vi "ControllerTestBench.vi"() -> ()   [LabVIEW 2016]
uses:
  <vilib>/addons/control/pid/pid.llb/PID (DBL).vi
  <vilib>/addons/Fuzzy Logic/FL Fuzzy Controller (MISO).vi
  <vilib>/addons/control/pid/NI_PID_pid.lvlib
  <vilib>/addons/Fuzzy Logic/NI_Fuzzy_Logic_API.lvlib
  <vilib>/Analysis/NI_AALBase.lvlib
panel:
  out "D":dbl
  out "I":dbl
  out "P":dbl
  out "v":dbl
  in  "RC out":dbl
  out "standard deviation":dbl format="%0.2f"
  out "mean":dbl format="%0.2f"
  out "Array":u32[](array[numeric])
  in  "Controller":enum16{"LQR", "Fuzzy", "P", "PD"}(ring)
  out "Output LQR":dbl
  out "LQR Direction":bool
  out "Fuzzy out":dbl
  in  "K":dbl[](array[numeric]) format="%#_13g"
  in  "Output range  P":cluster{"output high":dbl, "output low":dbl}={"output high"=100.0, "output low"=-100.0} {"output low" format="%.2f"; "output high" format="%.2f"}
  in  "P gains":T1={"Proportional gain (Kc)"=2.0, "Integral time (Ti, min)"=0.0, "Derivative time (Td, min)"=0.0} {"Derivative time (Td, min)" format="%.4f"; "Integral time (Ti, min)" format="%.3f"; "Proportional gain (Kc)" format="%.3f"}
  out "P output":dbl format="%.2f"
  in  "Number of iterations":i32=10000
  in  "Output range  PD":cluster{"output high":dbl, "output low":dbl}={"output high"=100.0, "output low"=-100.0} {"output low" format="%.2f"; "output high" format="%.2f"}
  in  "PD gains":T1={"Proportional gain (Kc)"=2.0, "Integral time (Ti, min)"=0.0, "Derivative time (Td, min)"=0.0} {"Derivative time (Td, min)" format="%.4f"; "Integral time (Ti, min)" format="%.3f"; "Proportional gain (Kc)" format="%.3f"}
  out "PD output":dbl format="%.2f"
  out "Elapsed time(usec)":dbl
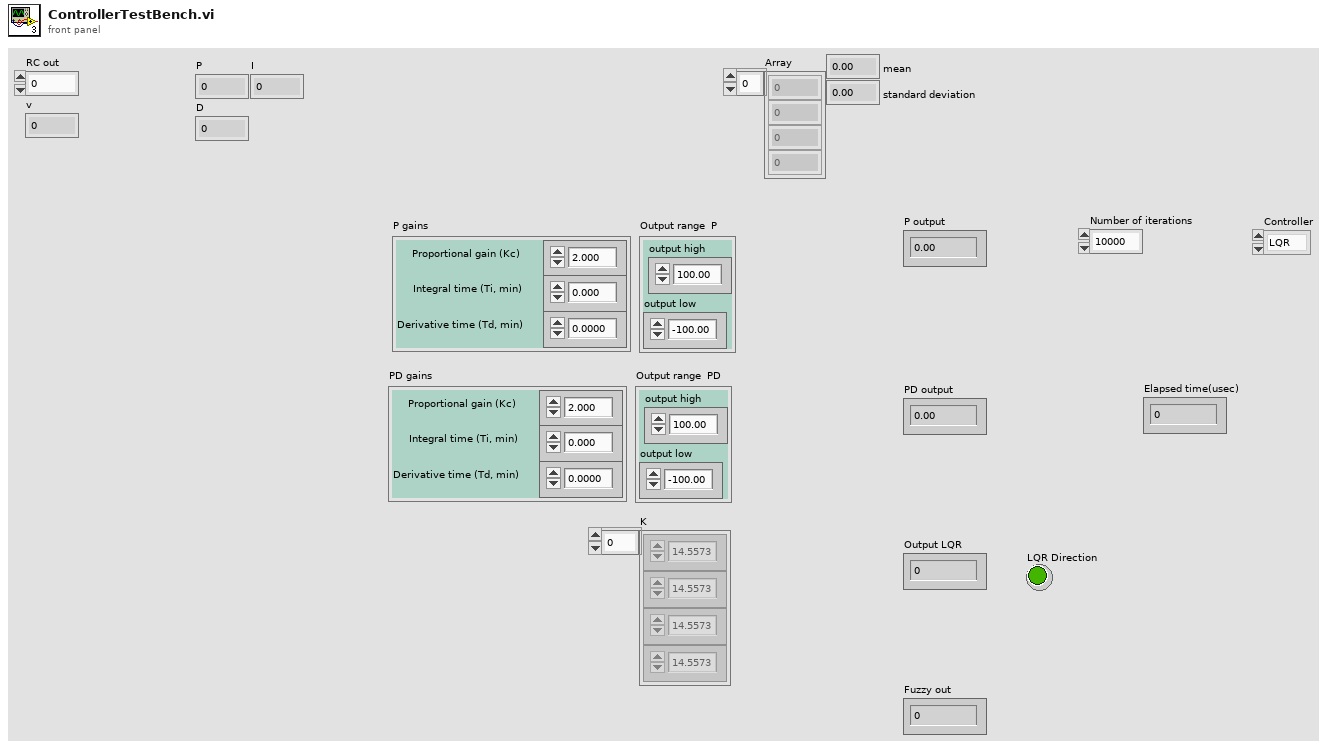
[diagram p1: front panel]
types:
  T1 = cluster{"Proportional gain (Kc)":dbl, "Integral time (Ti, min)":dbl, "Derivative time (Td, min)":dbl}
  T2 = typedef "NI_Fuzzy_Logic_API.lvlib/FL System.ctl" = cluster{"input variables":T3[], "output variables":T3[], "rules":T6[], "defuzzification method":T12, "description":string, "user MF interpolating polynomials":T13[]}
  T3 = typedef "NI_Fuzzy_Logic_API.lvlib/FL Variable.ctl" = cluster{"name":string, "range":dbl[], "MFs":T4[]}
  T4 = typedef "NI_Fuzzy_Logic_API.lvlib/FL Membership Function.ctl" = cluster{"name":string, "shape":T5, "points":dbl[], "color":u32, "user-defined shape index":i32}
  T5 = typedef "NI_Fuzzy_Logic_API.lvlib/FL Membership Function Shape.ctl" = u16
  T6 = typedef "NI_Fuzzy_Logic_API.lvlib/FL Rule.ctl" = cluster{"antecedents":T7[], "antecedent connective":T9, "consequents":T10[], "consequent implication":T11, "degree of support":dbl}
  T7 = typedef "NI_Fuzzy_Logic_API.lvlib/FL Antecedent.ctl" = cluster{"Var Index":i32, "MF Index":i32, "Cond":T8}
  T8 = typedef "NI_Fuzzy_Logic_API.lvlib/FL Modifier.ctl" = u16
  T9 = typedef "NI_Fuzzy_Logic_API.lvlib/FL Antecedent Connective.ctl" = u16
  T10 = typedef "NI_Fuzzy_Logic_API.lvlib/FL Consequent.ctl" = cluster{"Var Index":i32, "MF Index":i32, "Cond":T8}
  T11 = typedef "NI_Fuzzy_Logic_API.lvlib/FL Consequent Implication.ctl" = u16
  T12 = typedef "NI_Fuzzy_Logic_API.lvlib/FL Defuzzification.ctl" = u16
  T13 = typedef "NI_Fuzzy_Logic_API.lvlib/FL Interpolating polynomials.ctl" = cluster{"X":dbl[], "Y":dbl[], "Y(x) coeff":dbl[][], "X(y) coeff":dbl[][], "Area(y) coeff":dbl[][], "coa_x(y) coeff":dbl[][]}
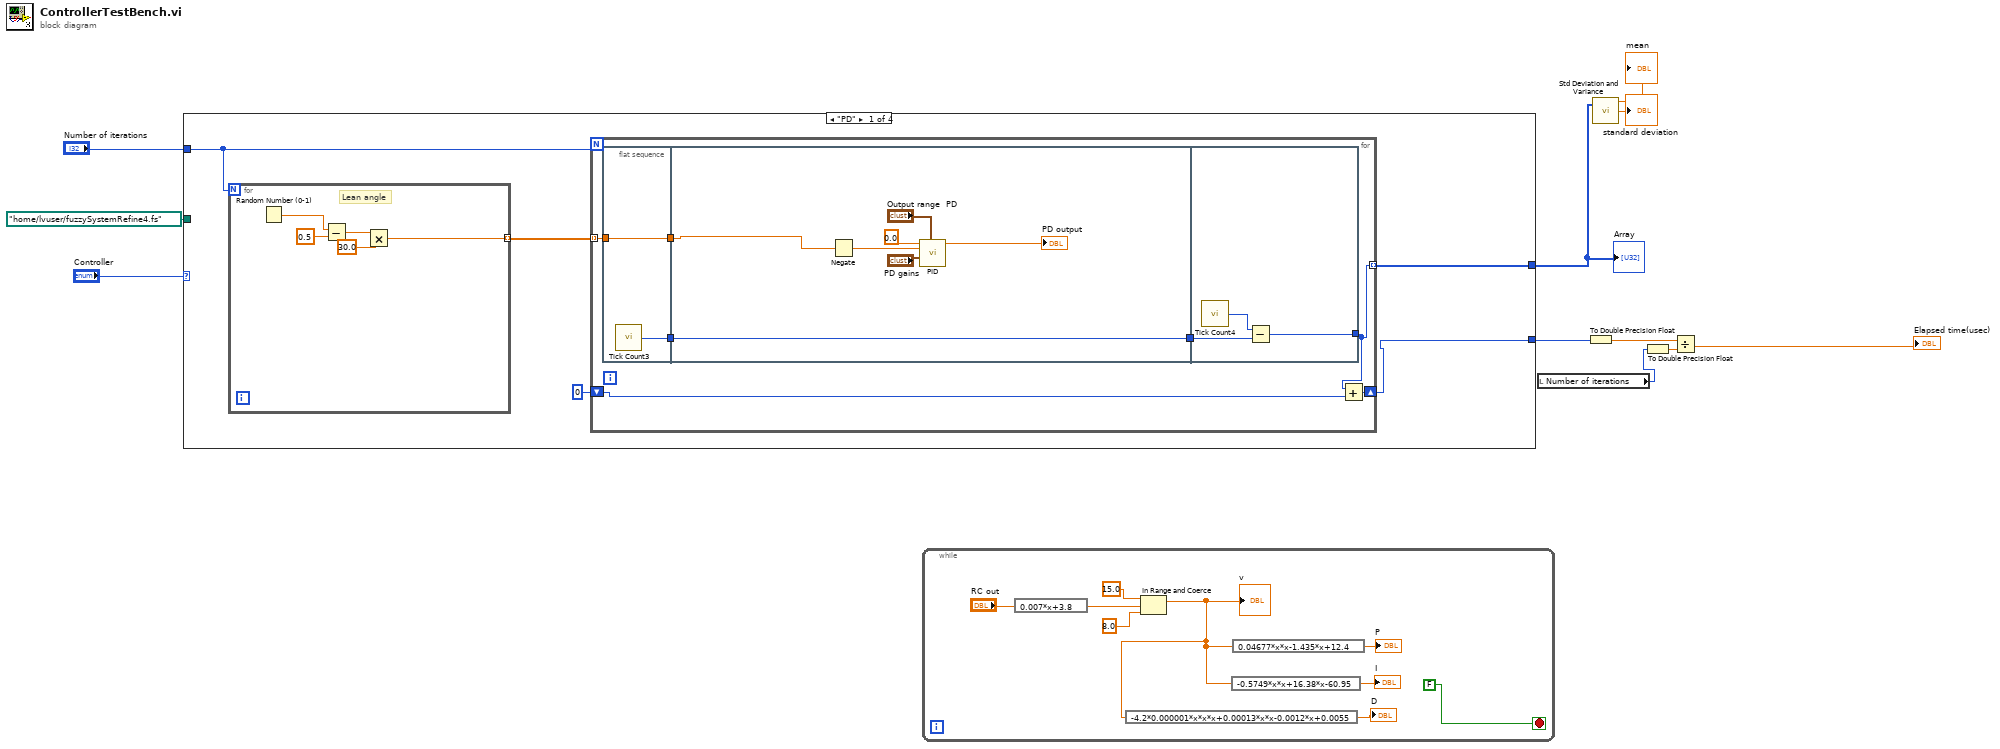
[diagram p0: block diagram]
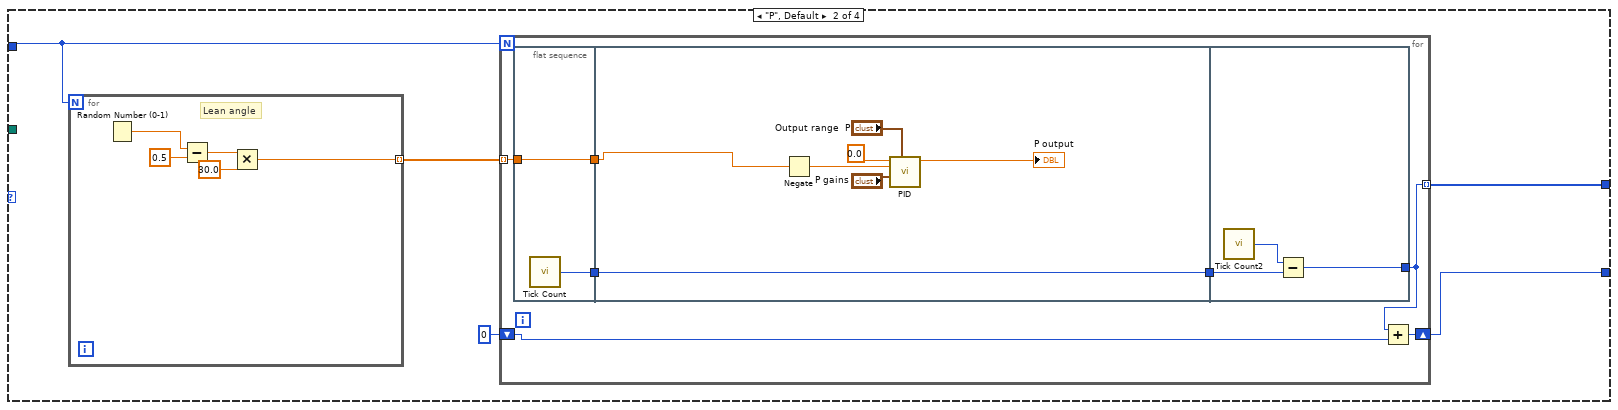
[diagram p2: hidden frame]
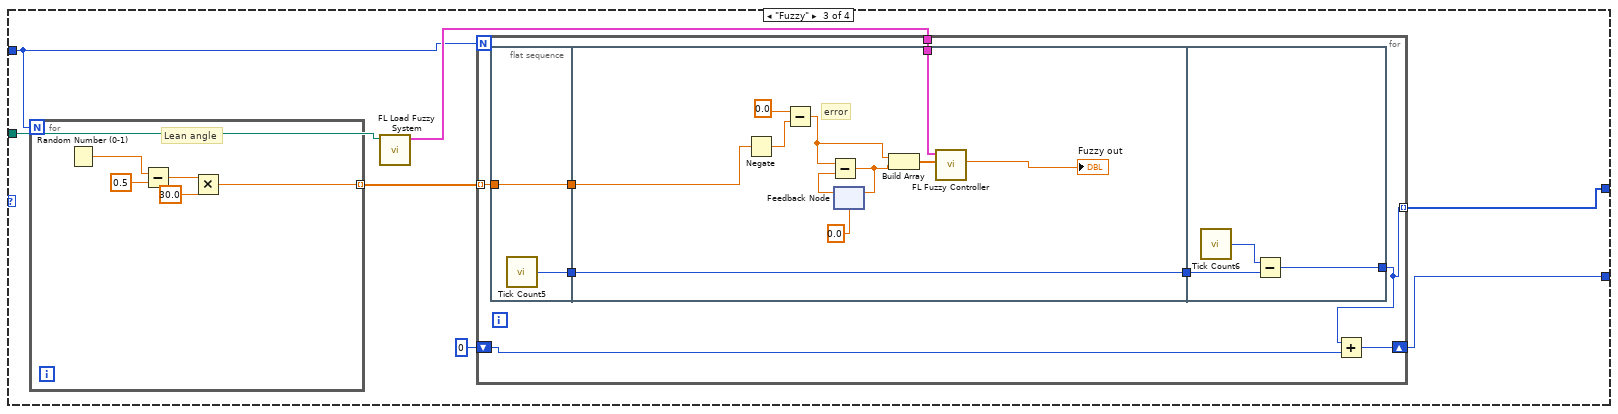
[diagram p3: hidden frame]
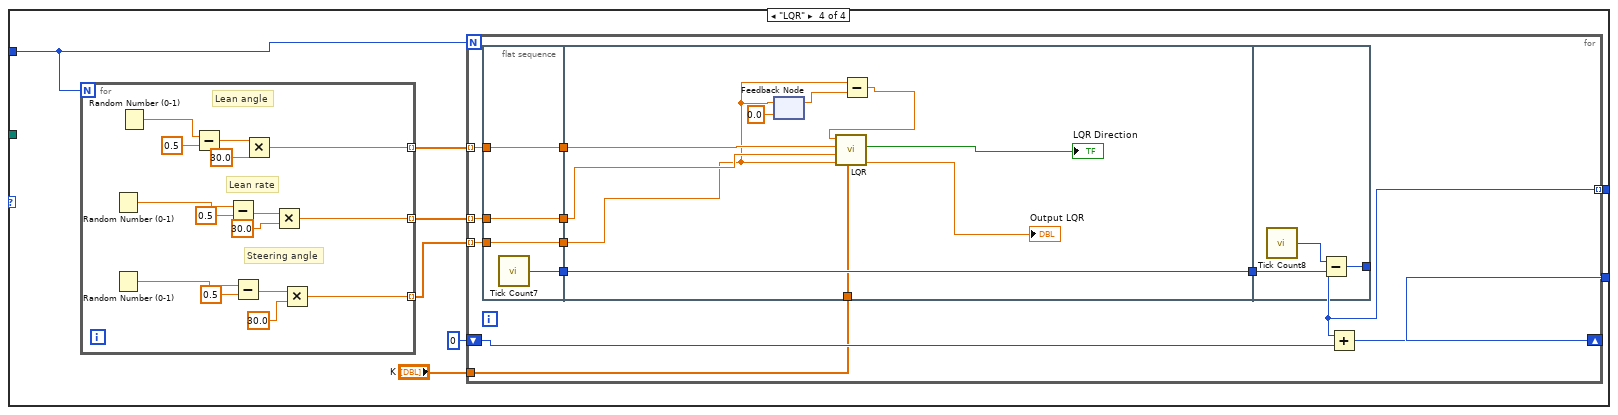
[diagram p4: hidden frame]
diagram:
  n1 = case shown="\"PD\"" "Controller" {
    tunnel: "Number of iterations" -> [w13 w42 w71 w111]
    tunnel: path "/home/lvuser/fuzzySystemRefine4.fs" ("file path") -> [_ _ w75 _]
    tunnel: [w15 w45 w73 w112] -> w5
    tunnel: [w12 w41 w70 w106] -> w3
    frame "PD" {
      n2 = for {
        N: w13 -> [_]
        tunnel: [w17] -> w14 mode=indexing
        # "Lean angle"
        n3 = Random Number (0-1)() -> (number: 0 to 1=w21:dbl)
        n4 = Subtract(x=w21, y=0.5) -> (x-y=w19:dbl)
        n5 = Multiply(x=w19, y=30.0) -> (x*y=w17:dbl)
      }
      n6 = for {
        N: w13 -> [_]
        shift-right: [w26] -> w15
        shift-left: u32 0 -> [w25]
        tunnel: w14 -> [w24] mode=indexing
        tunnel: [w22] -> w12 mode=indexing
        n7 = flat-sequence {
          tunnel: [w30] -> w27
          tunnel: w24 -> [w29]
          tunnel: [w29] -> w23
          tunnel: [w37] -> w28
          tunnel: w27 -> [w37]
          tunnel: w23 -> [w31]
          tunnel: w28 -> [w39]
          tunnel: [w38] -> w22
          frame #0 {
            n8 = call "Tick Count3"() -> ("Tick Count(uSec)"=w30:u32)
          }
          frame #1 {
            n9 = Negate(x=w31) -> (-x=w36:dbl)
            n10 = call-poly <vilib>:"PID.vi"("output range"="Output range  PD", "PID gains"="PD gains", "process variable"=w36, "setpoint"=0.0) -> ("output"=→"PD output":dbl)  [unwired: 6 in, 1 out]
          }
          frame #2 {
            n11 = call "Tick Count4"() -> ("Tick Count(uSec)"=w40:u32)
            n12 = Subtract(x=w40, y=w39) -> (x-y=w38:u32)
          }
        }
        n13 = Add(x=w22, y=w25) -> (x+y=w26:u32)
      }
    }
    frame "P", Default {
      n14 = for {
        N: w42 -> [_]
        tunnel: [w46] -> w43 mode=indexing
        # "Lean angle"
        n15 = Random Number (0-1)() -> (number: 0 to 1=w50:dbl)
        n16 = Subtract(x=w50, y=0.5) -> (x-y=w48:dbl)
        n17 = Multiply(x=w48, y=30.0) -> (x*y=w46:dbl)
      }
      n18 = for {
        N: w42 -> [_]
        shift-right: [w55] -> w45
        shift-left: u32 0 -> [w54]
        tunnel: w43 -> [w52] mode=indexing
        tunnel: [w51] -> w41 mode=indexing
        n19 = flat-sequence {
          tunnel: [w59] -> w56
          tunnel: [w58] -> w53
          tunnel: w52 -> [w58]
          tunnel: [w66] -> w57
          tunnel: w56 -> [w66]
          tunnel: w53 -> [w60]
          tunnel: w57 -> [w68]
          tunnel: [w67] -> w51
          frame #0 {
            n20 = call "Tick Count"() -> ("Tick Count(uSec)"=w59:u32)
          }
          frame #1 {
            n21 = Negate(x=w60) -> (-x=w65:dbl)
            n22 = call-poly <vilib>:"PID.vi"("output range"="Output range  P", "PID gains"="P gains", "process variable"=w65, "setpoint"=0.0) -> ("output"=→"P output":dbl)  [unwired: 6 in, 1 out]
          }
          frame #2 {
            n23 = call "Tick Count2"() -> ("Tick Count(uSec)"=w69:u32)
            n24 = Subtract(x=w69, y=w68) -> (x-y=w67:u32)
          }
        }
        n25 = Add(x=w51, y=w54) -> (x+y=w55:u32)
      }
    }
    frame "Fuzzy" {
      n26 = for {
        N: w71 -> [_]
        tunnel: [w77] -> w72 mode=indexing
        # "Lean angle"
        n27 = Random Number (0-1)() -> (number: 0 to 1=w81:dbl)
        n28 = Subtract(x=w81, y=0.5) -> (x-y=w79:dbl)
        n29 = Multiply(x=w79, y=30.0) -> (x*y=w77:dbl)
      }
      n30 = call <vilib>:"FL Load Fuzzy System.vi"("file path"=w75) -> ("fuzzy system out"=w76:T2)  [unwired: 9 in, 1 out]
      n31 = for {
        N: w71 -> [_]
        tunnel: w76 -> [w87]
        shift-right: [w86] -> w73
        shift-left: u32 0 -> [w85]
        tunnel: w72 -> [w83] mode=indexing
        tunnel: [w82] -> w70 mode=indexing
        n32 = flat-sequence {
          tunnel: [w91] -> w88
          tunnel: [w90] -> w84
          tunnel: w83 -> [w90]
          tunnel: [w102] -> w89
          tunnel: w88 -> [w102]
          tunnel: w87 -> [w93]
          tunnel: w84 -> [w92]
          tunnel: w89 -> [w104]
          tunnel: [w103] -> w82
          frame #0 {
            n33 = call "Tick Count5"() -> ("Tick Count(uSec)"=w91:u32)
          }
          frame #1 {
            # "error"
            n34 = Negate(x=w92) -> (-x=w101:dbl)
            n35 = Subtract(x=0.0 ("y"), y=w101) -> (x-y=w99:dbl)
            n36 = feedback #1(0.0 ("Lean Angle")) -> (w98:dbl)
            n37 = Subtract(x=w99, y=w98) -> (x-y=w100:dbl)
            n38 = feedback-in #1(w100) -> ()
            n39 = Build Array(w99, w100) -> (w96:dbl[])
            n40 = call-poly <vilib>:"FL Fuzzy Controller.vi"("input values"=w96, "fuzzy system in"=w93) -> ("output value"=→"Fuzzy out":dbl)  [unwired: 5 in, 4 out]
          }
          frame #2 {
            n41 = call "Tick Count6"() -> ("Tick Count(uSec)"=w105:u32)
            n42 = Subtract(x=w105, y=w104) -> (x-y=w103:u32)
          }
        }
        n43 = Add(x=w82, y=w85) -> (x+y=w86:u32)
      }
    }
    frame "LQR" {
      n44 = for {
        N: w111 -> [_]
        tunnel: [w116] -> w110 mode=indexing
        tunnel: [w115] -> w109 mode=indexing
        tunnel: [w114] -> w108 mode=indexing
        # "Steering angle"
        # "Lean rate"
        # "Lean angle"
        n45 = Random Number (0-1)() -> (number: 0 to 1=w123:dbl)
        n46 = Random Number (0-1)() -> (number: 0 to 1=w124:dbl)
        n47 = Random Number (0-1)() -> (number: 0 to 1=w128:dbl)
        n48 = Subtract(x=w128, y=0.5) -> (x-y=w126:dbl)
        n49 = Subtract(x=w123, y=0.5) -> (x-y=w120:dbl)
        n50 = Subtract(x=w124, y=0.5) -> (x-y=w119:dbl)
        n51 = Multiply(x=w126, y=30.0) -> (x*y=w116:dbl)
        n52 = Multiply(x=w120, y=30.0) -> (x*y=w115:dbl)
        n53 = Multiply(x=w119, y=30.0) -> (x*y=w114:dbl)
      }
      n54 = for {
        N: w111 -> [_]
        shift-right: [w138] -> w112
        shift-left: u32 0 -> [w137]
        tunnel: w110 -> [w136] mode=indexing
        tunnel: w109 -> [w134] mode=indexing
        tunnel: w108 -> [w132] mode=indexing
        tunnel: "K" -> [w130]
        tunnel: [w129] -> w106 mode=indexing
        n55 = flat-sequence {
          tunnel: [w144] -> w139
          tunnel: w136 -> [w143]
          tunnel: [w143] -> w135
          tunnel: w134 -> [w142]
          tunnel: [w142] -> w133
          tunnel: w132 -> [w141]
          tunnel: [w141] -> w131
          tunnel: [w154] -> w140
          tunnel: w139 -> [w154]
          tunnel: w135 -> [w148]
          tunnel: w133 -> [w147]
          tunnel: w131 -> [w146]
          tunnel: w130 -> [w145]
          tunnel: w140 -> [w156]
          tunnel: [w155] -> w129
          frame #0 {
            n56 = call "Tick Count7"() -> ("Tick Count(uSec)"=w144:u32)
          }
          frame #1 {
            n57 = feedback-in #2(w146) -> ()
            n58 = feedback #2(0.0 ("Steering angle in")) -> (w150:dbl)
            n59 = Subtract(x=w146, y=w150) -> (x-y=w151:dbl)
            n60 = call "LQR.vi"("K"=w145, "Steering angle in"=w146, "Lean rate in"=w147, "Lean angle in"=w148, "Steering rate"=w151) -> ("Duty cycle"=→"Output LQR":dbl, "Direction"=→"LQR Direction":bool)  [unwired: 4 in, 1 out]
          }
          frame #2 {
            n61 = call "Tick Count8"() -> ("Tick Count(uSec)"=w157:u32)
            n62 = Subtract(x=w157, y=w156) -> (x-y=w155:u32)
          }
        }
        n63 = Add(x=w129, y=w137) -> (x+y=w138:u32)
      }
    }
  }
  "Array" <- w3
  n64 = while {
    stop <- FALSE stop-if-true
    n65 = expression code="0.007*x+3.8"("RC out") -> (w165:dbl)
    n66 = In Range and Coerce(upper limit=15.0, x=w165, lower limit=8.0) -> (coerced(x)=w158:dbl)  [unwired: 1 out]
    "v" <- w158
    n67 = expression code="-4.2*0.000001*x*x*x+0.00013*x*x-0.0012*x+0.0055"(w158) -> (→"D":dbl)
    n68 = expression code="-0.5749*x*x+16.38*x-60.95"(w158) -> (→"I":dbl)
    n69 = expression code="0.04677*x*x-1.435*x+12.4"(w158) -> (→"P":dbl)
  }
  n70 = local read "Number of iterations"() -> (w7:i32)
  n71 = To Double Precision Float(number=w5) -> (double precision float=w10:dbl)
  n72 = call <vilib>:"Std Deviation and Variance.vi"("X"=w3) -> ("mean"=→"mean":dbl, "standard deviation"=→"standard deviation":dbl)  [unwired: 1 in, 1 out]
  n73 = To Double Precision Float(number=w7) -> (double precision float=w8:dbl)
  n74 = Divide(x=w10, y=w8) -> (x/y=→"Elapsed time(usec)":dbl)
